vi "SwerveDrivePoseEst2_InterpRecord_Interp.vi"(6 "Extra":variant, 9 "Time Fraction":dbl, 10 "End Input 2":variant, 11 "Input 1":variant) -> (3 "Interp Output":variant)   [LabVIEW 2019, in "Trajectory_Library.lvlib"]
doc: "Performs interpolation for a SwerveDrivePoseEstimator2 Interpolation Record.\n\nThis is an internal routine. It should NOT be used by end users."
uses:
  Trajectory_Library.lvlib
  TypeDef/SWERVE_DRIVE_KINEMATICS.ctl
  <vilib>/Analysis/Matrix/Datatypes/RealMatrix.ctl
  TypeDef/TRANSLATION2D.ctl
  TypeDef/SWERVE_DRIVE_MODULE_STATE.ctl
  TypeDef/ROTATION2D.ctl
  Rotation2d_Plus.vi
  MathUtil_Clamp.vi
  Rotation2d_Times.vi
  Rotation2d_UnaryMinus.vi
  Rotation2d_RotateBy.vi
  Rotation2d_CreateAngle.vi
  Rotation2d_CreateXY.vi
  Util_CalcDist.vi
  <vilib>/Analysis/Matrix/NI_Matrix.lvlib
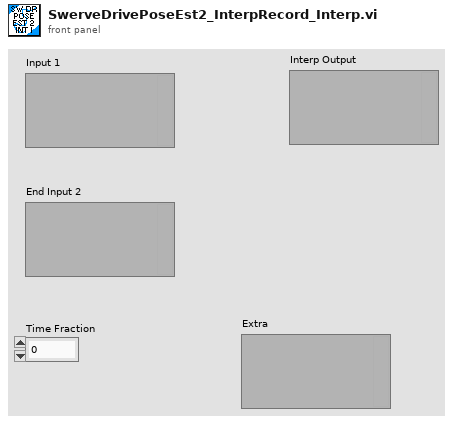
[diagram p1: front panel]
types:
  T1 = typedef "Trajectory_Library.lvlib/SWERVE_DRIVE_POSE_EST2_INTERP_RECORD.ctl" = cluster{"PoseMeters":T2, "GyroAngle":T4, "ModulePositions":T5[]}
  T2 = typedef "Trajectory_Library.lvlib/POSE2D.ctl" = cluster{"TRANSLATION":T3, "ROTATION":T4}
  T3 = typedef "Trajectory_Library.lvlib/TRANSLATION2D.ctl" = cluster{"X":dbl, "Y":dbl}
  T4 = typedef "Trajectory_Library.lvlib/ROTATION2D.ctl" = cluster{"VALUE":dbl, "COS":dbl, "SIN":dbl}
  T5 = typedef "Trajectory_Library.lvlib/SWERVE_DRIVE_MODULE_POSITION.ctl" = cluster{"Distance":dbl, "Angle":T4, "P":bool}
  T6 = typedef "Trajectory_Library.lvlib/SWERVE_DRIVE_KINEMATICS.ctl" = cluster{"NumModules":i32, "InverseKinematics":T7, "ForwardKinematics":T7, "Modules":T3[], "PrevCoR":T3, "SavedModuleStates":T8[]}
  T7 = typedef "NI_Matrix.lvlib/RealMatrix.ctl" = dbl[][]
  T8 = typedef "Trajectory_Library.lvlib/SWERVE_DRIVE_MODULE_STATE.ctl" = cluster{"Speed":dbl, "Angle":T4}
  T9 = typedef "Trajectory_Library.lvlib/TWIST2D.ctl" = cluster{"dX":dbl, "dY":dbl, "dTHETA":dbl}
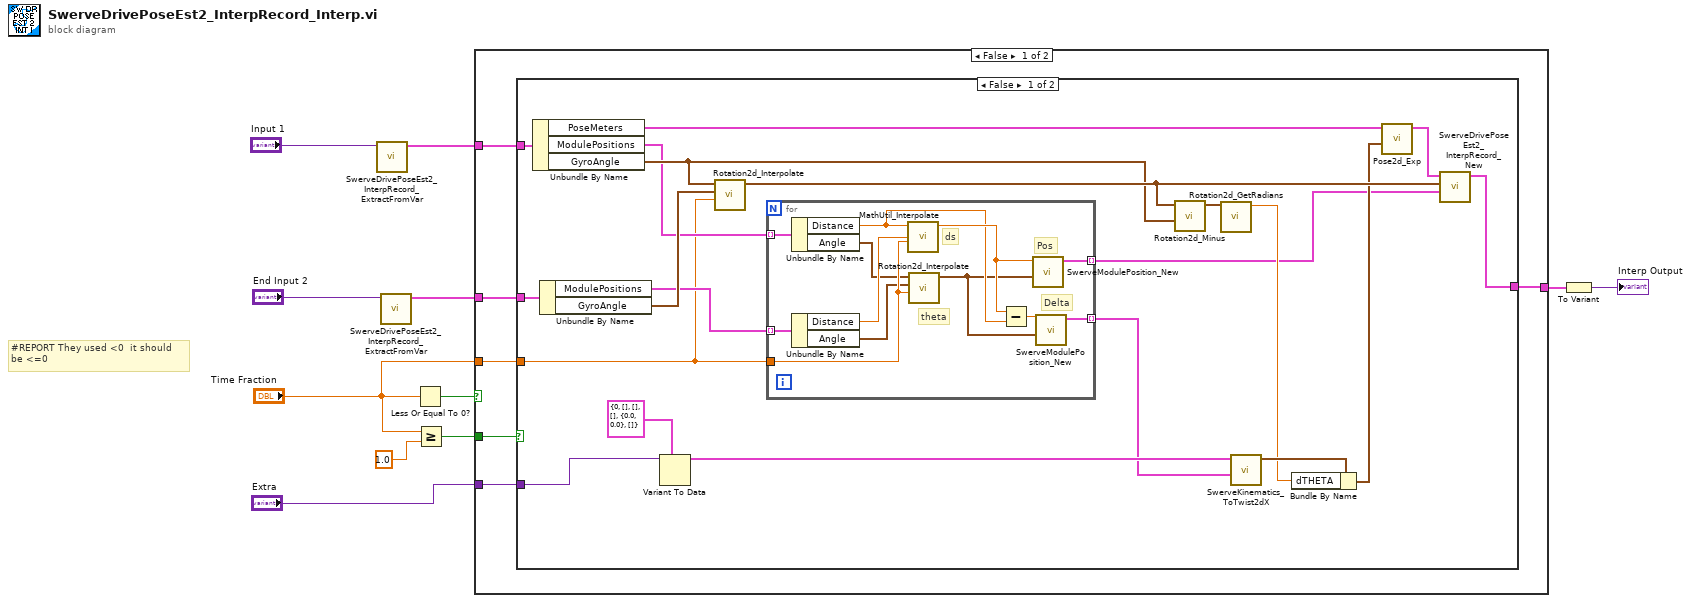
[diagram p0: block diagram]
diagram:
  # "#REPORT They used <0  it should\nbe <=0"
  n1 = call "SwerveDrivePoseEst2_InterpRecord_ExtractFromVar.vi"("OutputVariant"="Input 1") -> ("out InterpRecord"=w3:T1)  [unwired: 9 in, 1 out]
  n2 = call "SwerveDrivePoseEst2_InterpRecord_ExtractFromVar.vi"("OutputVariant"="End Input 2") -> ("out InterpRecord"=w1:T1)  [unwired: 9 in, 1 out]
  n3 = Less Or Equal To 0?(x="Time Fraction") -> (x <= 0?=w11:bool)
  n4 = Greater Or Equal?(x="Time Fraction", y=1.0) -> (x >= y?=w7:bool)
  n5 = case shown="False" w11 {
    tunnel: [w16 w51] -> w9
    tunnel: w3 -> [w14 w51]
    tunnel: w7 -> [w17 _]
    tunnel: w1 -> [w15 _]
    tunnel: "Time Fraction" -> [w13 _]
    tunnel: "Extra" -> [w12 _]
    frame False {
      n6 = case shown="False" w17 {
        tunnel: [w23 w50] -> w16
        tunnel: w15 -> [w36 w50]
        tunnel: w14 -> [w37 _]
        tunnel: w13 -> [w20 _]
        tunnel: w12 -> [w34 _]
        frame False {
          n7 = Unbundle By Name(w37) -> ("PoseMeters"=w26:T2, "ModulePositions"=w22:T5[], "GyroAngle"=w29:T4)
          n8 = Unbundle By Name(w36) -> ("ModulePositions"=w21:T5[], "GyroAngle"=w35:T4)
          n9 = Variant To Data(type=T6 {"NumModules"=0, "InverseKinematics"=[], "ForwardKinematics"=[], "Modules"=[], "PrevCoR"={"X"=0.0, "Y"=0.0}, "SavedModuleStates"=[]} ("SWERVE_DRIVE_KINEMATICS"), Variant=w34) -> (data=w32:T6)  [unwired: 1 in, 1 out]
          n10 = call "Rotation2d_Interpolate.vi"("T"=w20, "EncValue ROTATION"=w35, "in ROTATION"=w29) -> ("Interpolated ROTATION"=w30:T4)  [unwired: 8 in]
          n11 = for {
            tunnel: w22 -> [w49] mode=indexing
            tunnel: w21 -> [w48] mode=indexing
            tunnel: w20 -> [w46]
            tunnel: [w39] -> w18 mode=indexing
            tunnel: [w38] -> w19 mode=indexing
            # "Delta"
            # "Pos"
            # "theta"
            # "ds"
            n12 = Unbundle By Name(w49) -> ("Distance"=w41:dbl, "Angle"=w45:T4)
            n13 = Unbundle By Name(w48) -> ("Distance"=w47:dbl, "Angle"=w44:T4)
            n14 = call "MathUtil_Interpolate.vi"("T"=w46, "EndValue"=w47, "StartValue"=w41) -> ("InterpolatedValue"=w42:dbl)  [unwired: 8 in]
            n15 = call "Rotation2d_Interpolate.vi"("T"=w46, "EncValue ROTATION"=w44, "in ROTATION"=w45) -> ("Interpolated ROTATION"=w40:T4)  [unwired: 8 in]
            n16 = Subtract(x=w42, y=w41) -> (x-y=w43:dbl)
            n17 = call "SwerveModulePosition_New.vi"("ROTATION"=w40, "Distance"=w42) -> ("SWERVE_DRIVE_MODULE_POSITION"=w39:T5)  [unwired: 9 in]
            n18 = call "SwerveModulePosition_New.vi"("ROTATION"=w40, "Distance"=w43) -> ("SWERVE_DRIVE_MODULE_POSITION"=w38:T5)  [unwired: 9 in]
          }
          n19 = call "Rotation2d_Minus.vi"("other ROTATION"=w29, "in ROTATION"=w30) -> ("out ROTATION"=w28:T4)  [unwired: 9 in]
          n20 = call "Rotation2d_GetRadians.vi"("in ROTATION"=w28) -> ("AngleRadians"=w27:dbl)  [unwired: 10 in]
          n21 = call "SwerveKinematics_ToTwist2dX.vi"("WheelDeltas"=w19, "in SWERVE_DRIVE_KINEMATICS"=w32) -> ("Twist2d"=w31:T9)  [unwired: 8 in, 1 out]
          n22 = Bundle By Name(cluster=w31, "dTHETA"=w27) -> (w24:T9)
          n23 = call "Pose2d_Exp.vi"("TWIST"=w24, "POSE"=w26) -> ("UpdatedPose"=w25:T2)  [unwired: 9 in]
          n24 = call "SwerveDrivePoseEst2_InterpRecord_New.vi"("ModulePositions"=w18, "GyroAngle"=w30, "M_POSE_Meters"=w25) -> ("SWERVE_DRIVE_POSE_EST2_INTERP_RECORD"=w23:T1)  [unwired: 8 in]
        }
        frame True {
        }
      }
    }
    frame True {
    }
  }
  n25 = To Variant(anything=w9) -> (Variant=→"Interp Output":variant)
